vi "TSLIN_Table.vi"(8 "错误输入（无错误）":errorcluster, 9 "DataBase_array":T1, 10 "LIN_Buffer":T2[](array[typedef]), 11 "LIN_Data Ref":refnum<vi>) -> (0 "错误输出":errorcluster)   [LabVIEW 2014]
uses:
  Typedef/TLibLIN.ctl
  DataBase/Typedef/CAN/TCANSignal.ctl
  DataBase/Typedef/LIN/TLINSignal.ctl
  DataBase/Typedef/FlexRay/TFlexRaySignal.ctl
  DataBase/Typedef/TDBSignalProperties.ctl
  DataBase/Typedef/TDBFrameProperties.ctl
  DataBase/Typedef/TDBECUProperties.ctl
  DataBase/Typedef/TDBProperties.ctl
  DataBase/Typedef/DataBase_array.ctl
  DataBase/Typedef/DataBase_array_index.ctl
types:
  T1 = typedef "DataBase_array_index.ctl" = refnum<vi>
  T2 = typedef "TLibLIN.ctl" = cluster{"Ch":u8, "Code":u8, "Properties":u8, "FDLC":u8, "ID":u8, "Checksum":u8, "FStaus":u8, "FTimeUS":u64, "FDatas":cluster{"value0":u8, "value 1":u8, "value 2":u8, "value 3":u8, "value 4":u8, "value 5":u8, "value 6":u8, "value 7":u8}}
  T3 = typedef "DataBase_array.ctl" = cluster{"db_properties":T4, "ECU_array":cluster{"TDBECUProperties":T5, "TX_Frame_array":cluster{"Frame_Properties":T6, "signal_array":T7[]}[], "RX_Frame_array":cluster{"Frame_Properties":T6, "signal_array":T7[]}[]}[]}[]
  T4 = typedef "TDBProperties.ctl" = cluster{"FDBIndex":i32, "FSignalCount":i32, "FFrameCount":i32, "FECUCount":i32, "FSupportedChannelMask":u64, "FName":cluster{"数值":u64, "数值 2":u64, "数值 3":u64, "数值 4":u64, "数值 5":u64, "数值 6":u64, "数值 7":u64, "数值 8":u64, "数值 9":u64, "数值 10":u64, "数值 11":u64, "数值 12":u64, "数值 13":u64, "数值 14":u64, "数值 15":u64, "数值 16":u64, "数值 17":u64, "数值 18":u64, "数值 19":u64, "数值 20":u64, "数值 21":u64, "数值 22":u64, "数值 23":u64, "数值 24":u64, "数值 25":u64, "数值 26":u64, "数值 27":u64, "数值 28":u64, "数值 29":u64, "数值 30":u64, "数值 31":u64, "数值 32":u64, "数值 33":u64, "数值 34":u64, "数值 35":u64, "数值 36":u64, "数值 37":u64, "数值 38":u64, "数值 39":u64, "数值 40":u64, "数值 41":u64, "数值 42":u64, "数值 43":u64, "数值 44":u64, "数值 45":u64, "数值 46":u64, "数值 47":u64, "数值 48":u64, "数值 49":u64, "数值 50":u64, "数值 51":u64, "数值 52":u64, "数值 53":u64, "数值 54":u64, "数值 55":u64, "数值 56":u64, "数值 57":u64, "数值 58":u64, "数值 59":u64, "数值 60":u64, "数值 61":u64, "数值 62":u64, "数值 63":u64, "数值 64":u64}, "FComment":cluster{"数值":u64, "数值 2":u64, "数值 3":u64, "数值 4":u64, "数值 5":u64, "数值 6":u64, "数值 7":u64, "数值 8":u64, "数值 9":u64, "数值 10":u64, "数值 11":u64, "数值 12":u64, "数值 13":u64, "数值 14":u64, "数值 15":u64, "数值 16":u64, "数值 17":u64, "数值 18":u64, "数值 19":u64, "数值 20":u64, "数值 21":u64, "数值 22":u64, "数值 23":u64, "数值 24":u64, "数值 25":u64, "数值 26":u64, "数值 27":u64, "数值 28":u64, "数值 29":u64, "数值 30":u64, "数值 31":u64, "数值 32":u64, "数值 33":u64, "数值 34":u64, "数值 35":u64, "数值 36":u64, "数值 37":u64, "数值 38":u64, "数值 39":u64, "数值 40":u64, "数值 41":u64, "数值 42":u64, "数值 43":u64, "数值 44":u64, "数值 45":u64, "数值 46":u64, "数值 47":u64, "数值 48":u64, "数值 49":u64, "数值 50":u64, "数值 51":u64, "数值 52":u64, "数值 53":u64, "数值 54":u64, "数值 55":u64, "数值 56":u64, "数值 57":u64, "数值 58":u64, "数值 59":u64, "数值 60":u64, "数值 61":u64, "数值 62":u64, "数值 63":u64, "数值 64":u64}, "FFlags":u32, "FDBId":u32}
  T5 = typedef "TDBECUProperties.ctl" = cluster{"FDBIndex":i32, "FECUIndex":i32, "FTxFrameCount":i32, "FRxFrameCount":i32, "FName":cluster{"数值":u64, "数值 2":u64, "数值 3":u64, "数值 4":u64, "数值 5":u64, "数值 6":u64, "数值 7":u64, "数值 8":u64, "数值 9":u64, "数值 10":u64, "数值 11":u64, "数值 12":u64, "数值 13":u64, "数值 14":u64, "数值 15":u64, "数值 16":u64, "数值 17":u64, "数值 18":u64, "数值 19":u64, "数值 20":u64, "数值 21":u64, "数值 22":u64, "数值 23":u64, "数值 24":u64, "数值 25":u64, "数值 26":u64, "数值 27":u64, "数值 28":u64, "数值 29":u64, "数值 30":u64, "数值 31":u64, "数值 32":u64, "数值 33":u64, "数值 34":u64, "数值 35":u64, "数值 36":u64, "数值 37":u64, "数值 38":u64, "数值 39":u64, "数值 40":u64, "数值 41":u64, "数值 42":u64, "数值 43":u64, "数值 44":u64, "数值 45":u64, "数值 46":u64, "数值 47":u64, "数值 48":u64, "数值 49":u64, "数值 50":u64, "数值 51":u64, "数值 52":u64, "数值 53":u64, "数值 54":u64, "数值 55":u64, "数值 56":u64, "数值 57":u64, "数值 58":u64, "数值 59":u64, "数值 60":u64, "数值 61":u64, "数值 62":u64, "数值 63":u64, "数值 64":u64}, "FComment":cluster{"数值":u64, "数值 2":u64, "数值 3":u64, "数值 4":u64, "数值 5":u64, "数值 6":u64, "数值 7":u64, "数值 8":u64, "数值 9":u64, "数值 10":u64, "数值 11":u64, "数值 12":u64, "数值 13":u64, "数值 14":u64, "数值 15":u64, "数值 16":u64, "数值 17":u64, "数值 18":u64, "数值 19":u64, "数值 20":u64, "数值 21":u64, "数值 22":u64, "数值 23":u64, "数值 24":u64, "数值 25":u64, "数值 26":u64, "数值 27":u64, "数值 28":u64, "数值 29":u64, "数值 30":u64, "数值 31":u64, "数值 32":u64, "数值 33":u64, "数值 34":u64, "数值 35":u64, "数值 36":u64, "数值 37":u64, "数值 38":u64, "数值 39":u64, "数值 40":u64, "数值 41":u64, "数值 42":u64, "数值 43":u64, "数值 44":u64, "数值 45":u64, "数值 46":u64, "数值 47":u64, "数值 48":u64, "数值 49":u64, "数值 50":u64, "数值 51":u64, "数值 52":u64, "数值 53":u64, "数值 54":u64, "数值 55":u64, "数值 56":u64, "数值 57":u64, "数值 58":u64, "数值 59":u64, "数值 60":u64, "数值 61":u64, "数值 62":u64, "数值 63":u64, "数值 64":u64}}
  T6 = typedef "TDBFrameProperties.ctl" = cluster{"FDBIndex":i32, "FECUIndex":i32, "FFrameIndex":i32, "FIsTx":u8, "FReserved1":u8, "FCycleTimeMs":u16, "TSignalType":i32, "FCANIsDataFrame":u8, "FCANIsStdFrame":u8, "FCANIsEdl":u8, "FCANIsBrs":u8, "FCANIdentifier":i32, "FCANDLC":i32, "FCANDataBytes":i32, "FLINIdentifier":i32, "FLINDLC":i32, "FFRChannelMask":u8, "FFRBaseCycle":u8, "FFRCycleRepetition":u8, "FFRIsStartupFrame":u8, "FFRSlotId":u16, "FFRDLC":u16, "FFRCycleMask":u64, "FSignalCount":i32, "FName":cluster{"数值":u64, "数值 2":u64, "数值 3":u64, "数值 4":u64, "数值 5":u64, "数值 6":u64, "数值 7":u64, "数值 8":u64, "数值 9":u64, "数值 10":u64, "数值 11":u64, "数值 12":u64, "数值 13":u64, "数值 14":u64, "数值 15":u64, "数值 16":u64, "数值 17":u64, "数值 18":u64, "数值 19":u64, "数值 20":u64, "数值 21":u64, "数值 22":u64, "数值 23":u64, "数值 24":u64, "数值 25":u64, "数值 26":u64, "数值 27":u64, "数值 28":u64, "数值 29":u64, "数值 30":u64, "数值 31":u64, "数值 32":u64, "数值 33":u64, "数值 34":u64, "数值 35":u64, "数值 36":u64, "数值 37":u64, "数值 38":u64, "数值 39":u64, "数值 40":u64, "数值 41":u64, "数值 42":u64, "数值 43":u64, "数值 44":u64, "数值 45":u64, "数值 46":u64, "数值 47":u64, "数值 48":u64, "数值 49":u64, "数值 50":u64, "数值 51":u64, "数值 52":u64, "数值 53":u64, "数值 54":u64, "数值 55":u64, "数值 56":u64, "数值 57":u64, "数值 58":u64, "数值 59":u64, "数值 60":u64, "数值 61":u64, "数值 62":u64, "数值 63":u64, "数值 64":u64}, "FComment":cluster{"数值":u64, "数值 2":u64, "数值 3":u64, "数值 4":u64, "数值 5":u64, "数值 6":u64, "数值 7":u64, "数值 8":u64, "数值 9":u64, "数值 10":u64, "数值 11":u64, "数值 12":u64, "数值 13":u64, "数值 14":u64, "数值 15":u64, "数值 16":u64, "数值 17":u64, "数值 18":u64, "数值 19":u64, "数值 20":u64, "数值 21":u64, "数值 22":u64, "数值 23":u64, "数值 24":u64, "数值 25":u64, "数值 26":u64, "数值 27":u64, "数值 28":u64, "数值 29":u64, "数值 30":u64, "数值 31":u64, "数值 32":u64, "数值 33":u64, "数值 34":u64, "数值 35":u64, "数值 36":u64, "数值 37":u64, "数值 38":u64, "数值 39":u64, "数值 40":u64, "数值 41":u64, "数值 42":u64, "数值 43":u64, "数值 44":u64, "数值 45":u64, "数值 46":u64, "数值 47":u64, "数值 48":u64, "数值 49":u64, "数值 50":u64, "数值 51":u64, "数值 52":u64, "数值 53":u64, "数值 54":u64, "数值 55":u64, "数值 56":u64, "数值 57":u64, "数值 58":u64, "数值 59":u64, "数值 60":u64, "数值 61":u64, "数值 62":u64, "数值 63":u64, "数值 64":u64}}
  T7 = typedef "TDBSignalProperties.ctl" = cluster{"FDBIndex":i32, "FECUIndex":i32, "FFrameIndex":i32, "FSignalIndex":i32, "FIsTx":u8, "FReserved1":u8, "FReserved2":u8, "FReserved3":u8, "TSignalType":i32, "TCANSignal":T8, "TLINSignal":T9, "TFlexRaySignal":T10, "FParentFrameId":i32, "FInitValue":dbl, "FName":cluster{"数值":u64, "数值 2":u64, "数值 3":u64, "数值 4":u64, "数值 5":u64, "数值 6":u64, "数值 7":u64, "数值 8":u64, "数值 9":u64, "数值 10":u64, "数值 11":u64, "数值 12":u64, "数值 13":u64, "数值 14":u64, "数值 15":u64, "数值 16":u64, "数值 17":u64, "数值 18":u64, "数值 19":u64, "数值 20":u64, "数值 21":u64, "数值 22":u64, "数值 23":u64, "数值 24":u64, "数值 25":u64, "数值 26":u64, "数值 27":u64, "数值 28":u64, "数值 29":u64, "数值 30":u64, "数值 31":u64, "数值 32":u64, "数值 33":u64, "数值 34":u64, "数值 35":u64, "数值 36":u64, "数值 37":u64, "数值 38":u64, "数值 39":u64, "数值 40":u64, "数值 41":u64, "数值 42":u64, "数值 43":u64, "数值 44":u64, "数值 45":u64, "数值 46":u64, "数值 47":u64, "数值 48":u64, "数值 49":u64, "数值 50":u64, "数值 51":u64, "数值 52":u64, "数值 53":u64, "数值 54":u64, "数值 55":u64, "数值 56":u64, "数值 57":u64, "数值 58":u64, "数值 59":u64, "数值 60":u64, "数值 61":u64, "数值 62":u64, "数值 63":u64, "数值 64":u64}, "FComment":cluster{"数值":u64, "数值 2":u64, "数值 3":u64, "数值 4":u64, "数值 5":u64, "数值 6":u64, "数值 7":u64, "数值 8":u64, "数值 9":u64, "数值 10":u64, "数值 11":u64, "数值 12":u64, "数值 13":u64, "数值 14":u64, "数值 15":u64, "数值 16":u64, "数值 17":u64, "数值 18":u64, "数值 19":u64, "数值 20":u64, "数值 21":u64, "数值 22":u64, "数值 23":u64, "数值 24":u64, "数值 25":u64, "数值 26":u64, "数值 27":u64, "数值 28":u64, "数值 29":u64, "数值 30":u64, "数值 31":u64, "数值 32":u64, "数值 33":u64, "数值 34":u64, "数值 35":u64, "数值 36":u64, "数值 37":u64, "数值 38":u64, "数值 39":u64, "数值 40":u64, "数值 41":u64, "数值 42":u64, "数值 43":u64, "数值 44":u64, "数值 45":u64, "数值 46":u64, "数值 47":u64, "数值 48":u64, "数值 49":u64, "数值 50":u64, "数值 51":u64, "数值 52":u64, "数值 53":u64, "数值 54":u64, "数值 55":u64, "数值 56":u64, "数值 57":u64, "数值 58":u64, "数值 59":u64, "数值 60":u64, "数值 61":u64, "数值 62":u64, "数值 63":u64, "数值 64":u64}}
  T8 = typedef "TCANSignal.ctl" = cluster{"FCANSgnType":u8, "FIsIntel":u8, "FStartBit":i32, "FLength":i32, "FFactor":dbl, "FOffset":dbl}
  T9 = typedef "TLINSignal.ctl" = cluster{"FLINSgnType":u8, "FIsIntel":u8, "FStartBit":i32, "FLength":i32, "FFactor":dbl, "FOffset":dbl}
  T10 = typedef "TFlexRaySignal.ctl" = cluster{"FFRSgnType":u8, "FCompuMethod":u8, "FReserved":u8, "FIsIntel":u8, "FStartBit":i32, "FUpdateBit":i32, "FLength":i32, "FFactor":dbl, "FOffset":dbl, "FActualStartBit":i32, "FActualUpdateBit":i32}
  T11 = cluster{"Message Name":string, "Signal Names":string[], "Signal_Values":dbl[]}
  T12 = cluster{"value0":u8, "value 1":u8, "value 2":u8, "value 3":u8, "value 4":u8, "value 5":u8, "value 6":u8, "value 7":u8}
  T13 = typedef "LVRowAndColumnUnsignedTypeDef.ctl" = cluster{"Row":u32, "Column":u32}
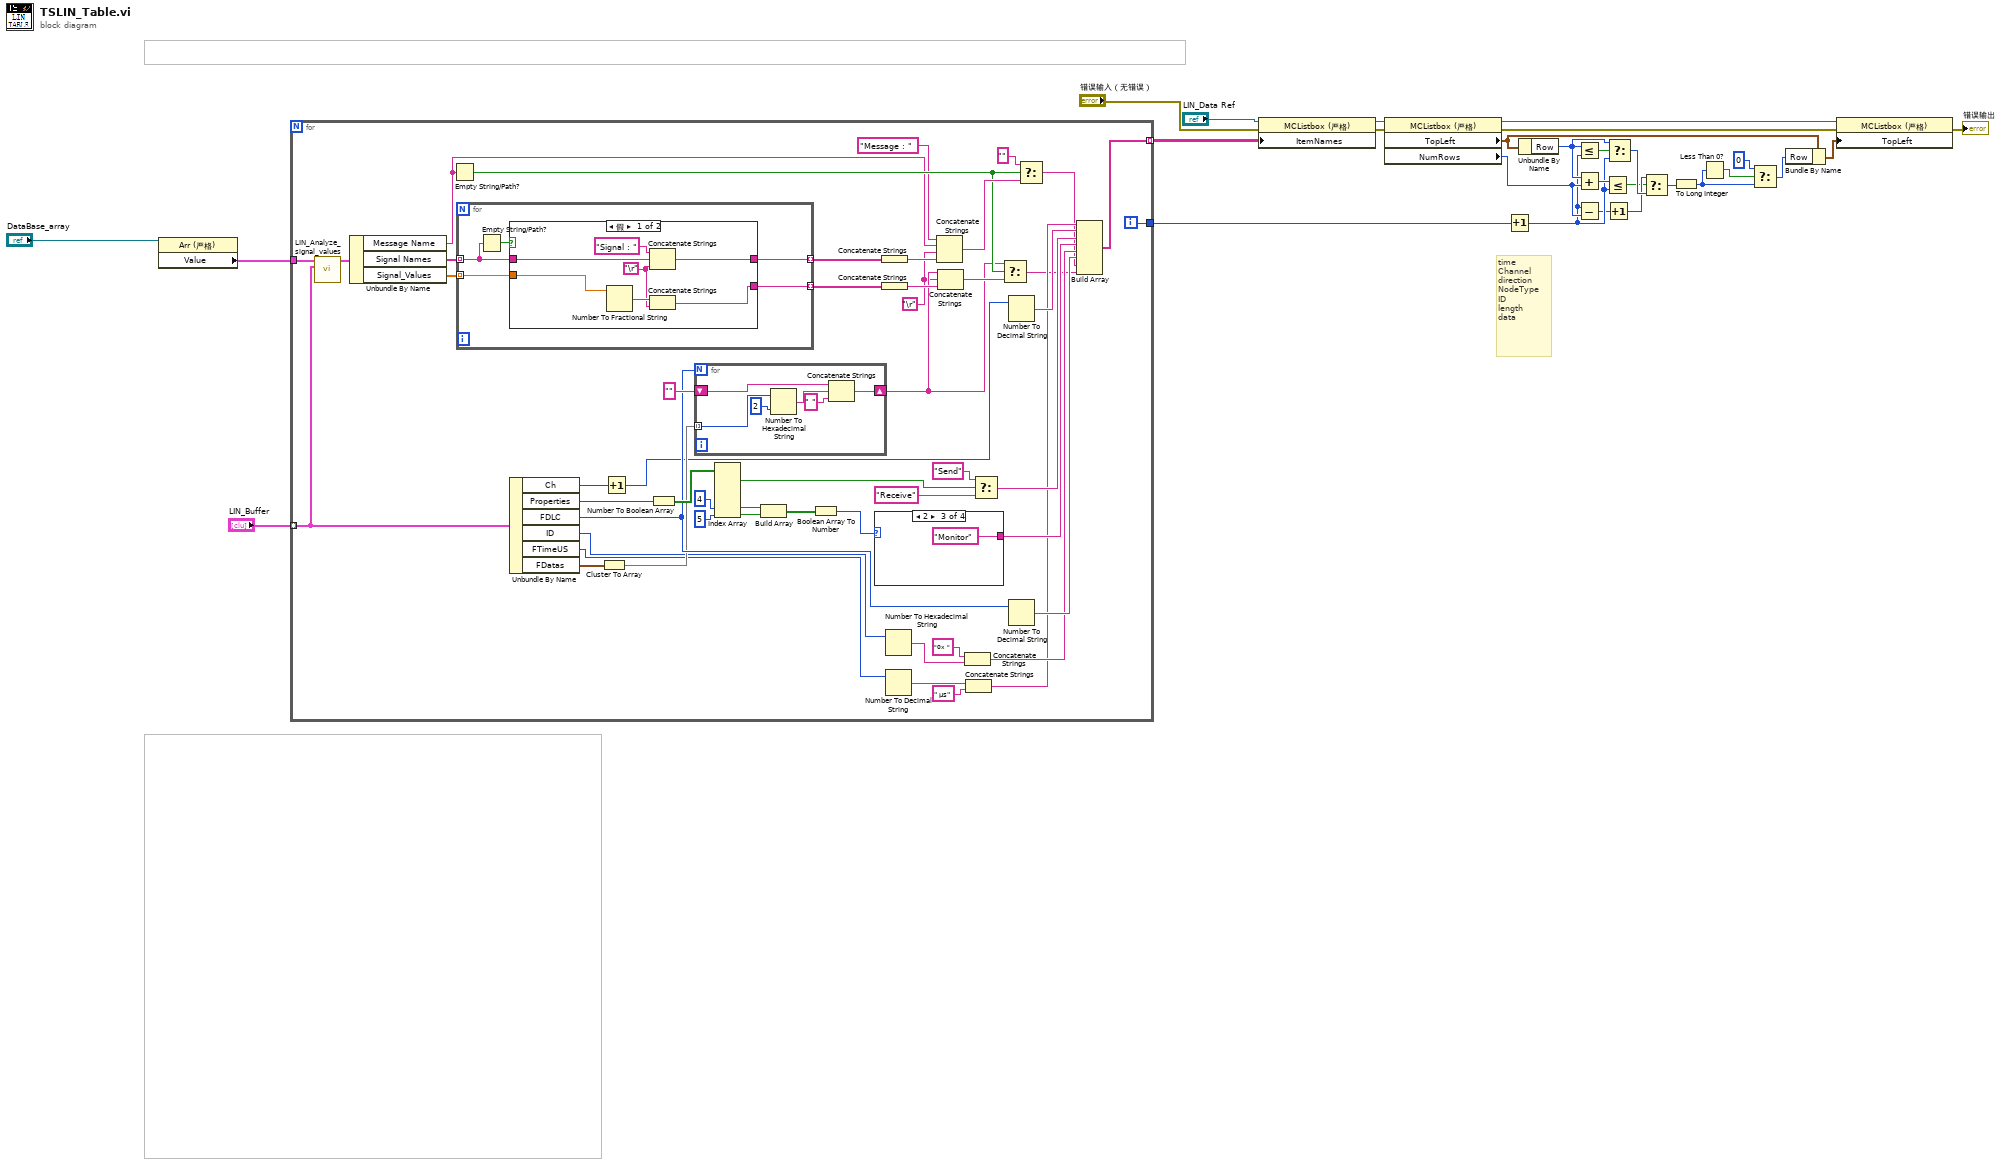
[diagram p0: block diagram]
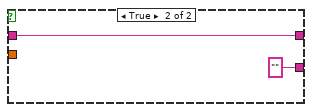
[diagram p2: hidden frame]
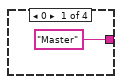
[diagram p3: hidden frame]
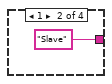
[diagram p4: hidden frame]
diagram:
  # "time\nChannel\ndirection\nNodeType\nID\nlength\ndata"
  n1 = property class="Arr (严格)"(reference="DataBase_array") -> ("Value"=w2:T3)  [unwired: 1 in, 2 out]
  n2 = for {
    tunnel: "LIN_Buffer" -> [w47] mode=indexing
    tunnel: [w66] -> w28 mode=indexing
    tunnel: [w52] -> w3
    tunnel: w2 -> [w46]
    i -> [w52]
    w29 = "\r"
    n3 = call "LIN_Analyze_signal_values.vi"("ALINData"=w47, "LDF_data_array"=w46) -> ("data out"=w45:T11)  [unwired: 9 in]
    n4 = Unbundle By Name(w45) -> ("Message Name"=w35:string, "Signal Names"=w44:string[], "Signal_Values"=w43:dbl[])
    n5 = Empty String/Path?(string/path=w35) -> (empty?=w38:bool)
    n6 = for {
      tunnel: w44 -> [w83] mode=indexing
      tunnel: [w82] -> w42 mode=indexing
      tunnel: w43 -> [w80] mode=indexing
      tunnel: [w79] -> w41 mode=indexing
      n7 = Empty String/Path?(string/path=w83) -> (empty?=w81:bool)
      n8 = case shown="假" w81 {
        tunnel: w83 -> [w90 w92]
        tunnel: [w89 w92] -> w82
        tunnel: w80 -> [w87 _]
        tunnel: [w84 ""] -> w79
        frame False {
          w85 = "\r"
          n9 = Number To Fractional String(number=w87) -> (F-format string=w86:string)  [unwired: 3 in]
          n10 = Concatenate Strings("Signal : " ("字符串"), w90, w85) -> (w89:string)
          n11 = Concatenate Strings(w86, w85) -> (w84:string)
        }
        frame True {
        }
      }
    }
    n12 = Unbundle By Name(w47) -> ("Ch"=w65:u8, "Properties"=w78:u8, "FDLC"=w72:u8, "ID"=w57:u8, "FTimeUS"=w51:u64, "FDatas"=w48:T12)
    n13 = Cluster To Array(cluster=w48) -> (array=w71:u8[])
    n14 = Increment(x=w65) -> (x+1=w64:u8)
    n15 = Number To Boolean Array(number=w78) -> (Boolean array=w77:bool[])
    n16 = for {
      N: w72 -> [_]
      tunnel: w71 -> [w98] mode=indexing
      shift-right: [w100] -> w30
      shift-left: "" -> [w101]
      n17 = Number To Hexadecimal String(1:i16 2 ("width (-)"), 2:w98) -> (0:w97:string)
      n18 = Concatenate Strings(w101, w97, " " ("string")) -> (w100:string)
    }
    n19 = Index Array(array=w77, index #5=4 ("索引"), index #6=5 ("索引")) -> (element #1=w76:bool, element #5=w56:bool, element #6=w55:bool)  [unwired: 4 in, 3 out]
    n20 = Build Array(w56, w55) -> (w54:bool[])
    n21 = Boolean Array To Number(Boolean array=w54) -> (number=w53:u32)
    n22 = case shown="2" w53 {
      tunnel: ["Master" "Slave" "Monitor" _] -> w68
      frame 0 {
      }
      frame 1 {
      }
      frame 2 {
      }
      frame 3, Default {
      }
    }
    n23 = Concatenate Strings(w42) -> (w34:string)
    n24 = Concatenate Strings(w41) -> (w33:string)
    n25 = Number To Hexadecimal String(2:w57) -> (0:w62:string)  [unwired: 1 in]
    n26 = Number To Decimal String(number=w51) -> (decimal integer string=w59:string)  [unwired: 1 in]
    n27 = Concatenate Strings("Message : " ("字符串"), w35, w29, w34) -> (w39:string)
    n28 = Concatenate Strings(w30, w29, w33) -> (w37:string)
    n29 = Concatenate Strings("0x " ("字符串"), w62) -> (w63:string)
    n30 = Concatenate Strings(w59, " μs" ("字符串")) -> (w60:string)
    n31 = Select(t="Send", s=w76, f="Receive") -> (s? t:f=w69:string)
    n32 = Select(t=w30, s=w38, f=w37) -> (s? t:f=w31:string)
    n33 = Number To Decimal String(number=w64) -> (decimal integer string=w70:string)  [unwired: 1 in]
    n34 = Number To Decimal String(number=w72) -> (decimal integer string=w67:string)  [unwired: 1 in]
    n35 = Select(t="", s=w38, f=w39) -> (s? t:f=w32:string)
    n36 = Build Array(w60, w70, w69, w68, w63, w67, w32, w31) -> (w66:string[])
  }
  n37 = property class="MCListbox (严格)"(reference="LIN_Data Ref", error in="错误输入（无错误）", "ItemNames"=w28) -> (reference out=w10:refnum<vi>, error out=w7:errorcluster)
  n38 = property class="MCListbox (严格)"(reference=w10, error in=w7) -> (reference out=w18:refnum<vi>, error out=w6:errorcluster, "TopLeft"=w17:T13, "NumRows"=w25:u32)
  n39 = Increment(x=w3) -> (x+1=w23:i32)
  n40 = Unbundle By Name(w17) -> ("Row"=w26:u32)
  n41 = Less Or Equal?(x=w26, y=w23) -> (x <= y?=w27:bool)
  n42 = Add(x=w26, y=w25) -> (x+y=w24:u32)
  n43 = Subtract(x=w23, y=w25) -> (x-y=w22:u32)
  n44 = Less Or Equal?(x=w24, y=w23) -> (x <= y?=w19:bool)
  n45 = Increment(x=w22) -> (x+1=w20:u32)
  n46 = Select(t=w26, s=w27, f=w23) -> (s? t:f=w21:u32)
  n47 = Select(t=w20, s=w19, f=w21) -> (s? t:f=w16:u32)
  n48 = To Long Integer(number=w16) -> (32bit integer=w14:i32)
  n49 = Less Than 0?(x=w14) -> (x < 0?=w15:bool)
  n50 = Select(t=0, s=w15, f=w14) -> (s? t:f=w13:i32)
  n51 = Bundle By Name(cluster=w17, "Row"=w13) -> (w11:T13)
  n52 = property class="MCListbox (严格)"(reference=w18, error in=w6, "TopLeft"=w11) -> (error out=→"错误输出":errorcluster)  [unwired: 1 out]
